vi "Minimize.vi"(8 "error in":errorcluster, 11 "Philips Subpanel in":refnum<class "Flex UI Subpanel.lvclass">) -> (0 "error out":errorcluster, 3 "Philips Subpanel out":refnum<class "Flex UI Subpanel.lvclass">)   [LabVIEW 2014, in "Flex UI Subpanel.lvclass"]
doc: "Minimizes the UI."
uses:
  Flex UI Subpanel.lvclass
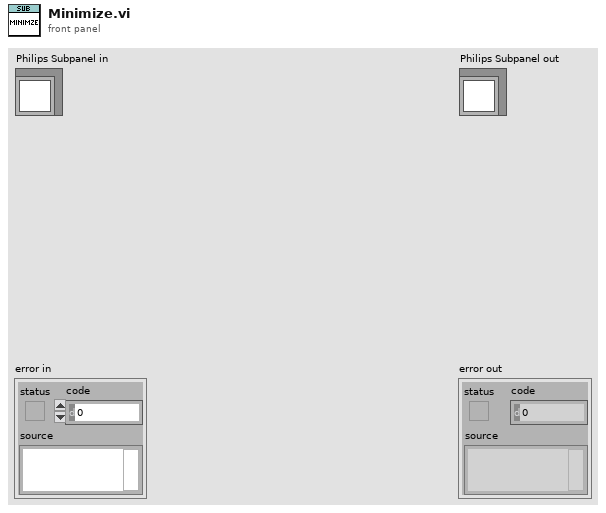
[diagram p1: front panel]
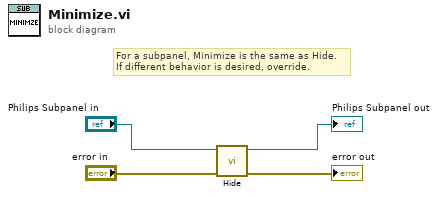
[diagram p0: block diagram]
diagram:
  # "For a subpanel, Minimize is the same as Hide.\nIf different behavior is desired, override."
  n1 = call-dynamic "Hide.vi"("error in"="error in", "Philips Subpanel in"="Philips Subpanel in") -> ("error out"=→"error out":errorcluster, "Philips Subpanel out"=→"Philips Subpanel out":refnum<class "Flex UI Subpanel.lvclass">)  [unwired: 8 in]
